vi "andor3test.vi"() -> ()   [LabVIEW 2010]
uses:
  <userlib>/Imaging/classes/AndorSDK3/AndorSDK3.lvclass
  <userlib>/Imaging/subvis/ExposureSettings.ctl
  <userlib>/Imaging/subvis/ROI_rect.ctl
panel:
  out "capturing?":bool
  out "error out":errorcluster
  out "attributes":variant[](array[variant])
  out "Graph":u16[][](graph)
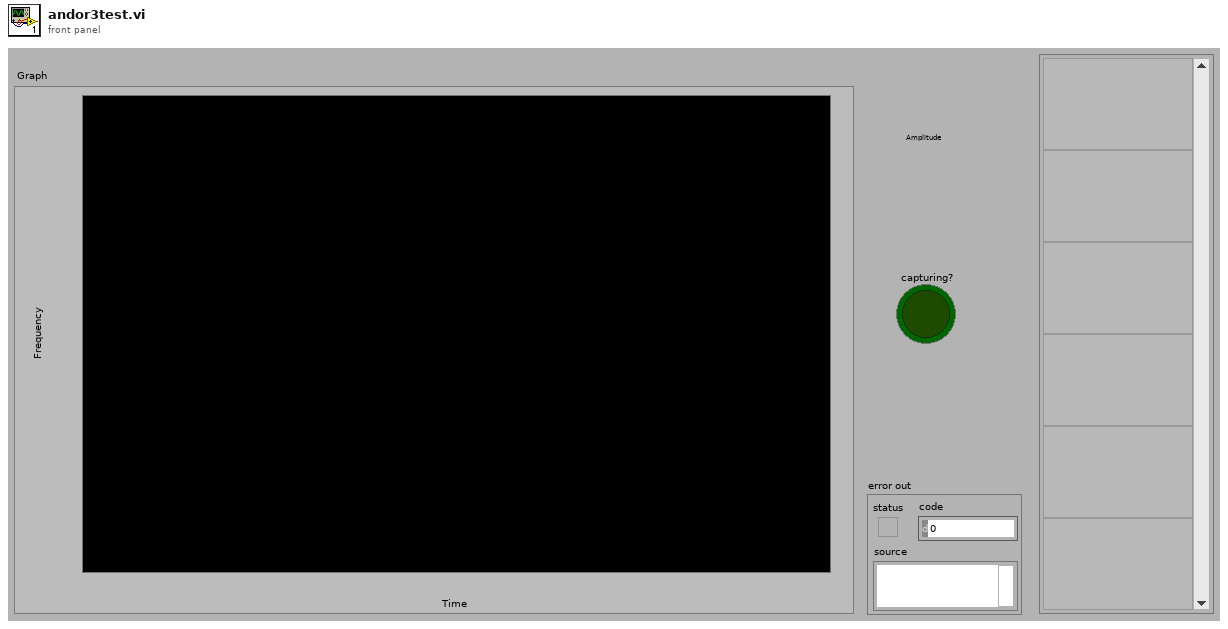
[diagram p1: front panel]
types:
  T1 = typedef "ExposureSettings.ctl" = cluster{"exposure":dbl, "external":bool, "roi":T2, "frames":i32, "bin_x":u8, "bin_y":u8}
  T2 = typedef "ROI_rect.ctl" = cluster{"left":i32, "top":i32, "right":i32, "bottom":i32}
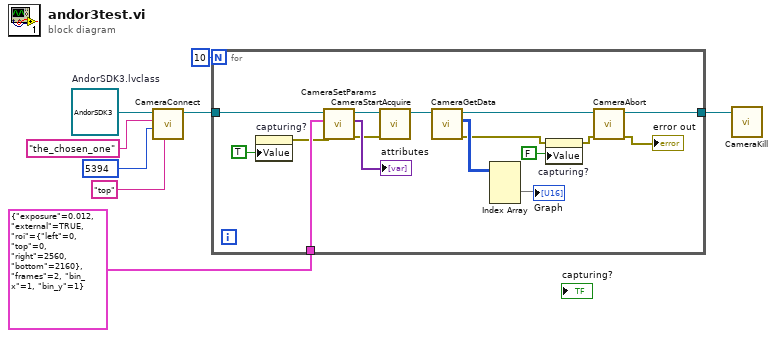
[diagram p0: block diagram]
diagram:
  w8 = refnum<class "AndorSDK3.lvclass"> refnum  # AndorSDK3.lvclass
  n1 = call-dynamic "CameraConnect.vi"("location"="top", "serial"=u64 5394, "name"="the_chosen_one", "AndorSDK3 in"=w8) -> ("AndorSDK3 out"=w4:refnum<class "AndorSDK3.lvclass">)  [unwired: 5 in, 2 out]
  n2 = for {
    N: 10 -> [_]
    tunnel: w4 -> [w24]
    tunnel: T1 {"exposure"=0.012, "external"=TRUE, "roi"={"left"=0, "top"=0, "right"=2560, "bottom"=2160}, "frames"=2, "bin_x"=1, "bin_y"=1} ("settings") -> [w21]
    tunnel: [w17] -> w2
    n3 = property on="capturing?" class="Bool (strict)"("Value"=TRUE ("Boolean")) -> (error out=w14:errorcluster)  [unwired: 2 in, 1 out]
    n4 = call-dynamic "CameraSetParams.vi"("error in (no error)"=w14, "settings"=w21, "AndorSDK3 in"=w24) -> ("error out"=w15:errorcluster, "attributes"=→"attributes":variant[], "AndorSDK3 out"=w23:refnum<class "AndorSDK3.lvclass">)  [unwired: 5 in, 1 out]
    n5 = call-dynamic "CameraStartAcquire.vi"("error in (no error)"=w15, "AndorSDK3 in"=w23) -> ("AndorSDK3 out"=w22:refnum<class "AndorSDK3.lvclass">)  [unwired: 8 in, 1 out]
    n6 = call-dynamic "CameraGetData.vi"("AndorSDK2 in"=w22) -> ("error out"=w9:errorcluster, "image_data"=w19:u16[][][], "AndorSDK2 out"=w20:refnum<class "AndorSDK3.lvclass">)  [unwired: 8 in]
    n7 = Index Array(array=w19) -> (element=→"Graph":u16[][])  [unwired: 3 in]
    n8 = property on="capturing?" class="Bool (strict)"(error in=w9, "Value"=FALSE ("Boolean")) -> (error out=w10:errorcluster)  [unwired: 1 in, 1 out]
    n9 = call-dynamic "CameraAbort.vi"("error in"=w10, "AndorSDK3 in"=w20) -> ("error out"=→"error out":errorcluster, "AndorSDK3 out"=w17:refnum<class "AndorSDK3.lvclass">)  [unwired: 8 in]
  }
  n10 = call-dynamic "CameraKill.vi"("AndorSDK3 in"=w2) -> ()  [unwired: 9 in, 2 out]
